vi "Lex Text-{} Unescaped Variable.vi"(8 "Error In":errorcluster) -> (0 "Error Out":errorcluster)   [LabVIEW 2018, in "Tests.lvlib" / "Lexer.lvlib"]
uses:
  Lexer.lvlib
  src/Toolkit/Low-Level/Tokens/Text/Text.lvclass
  src/Toolkit/Low-Level/Tokens/UnescapedVariable/UnescapedVariable.lvclass
  src/Toolkit/Low-Level/Tokens/Keyable/Keyable.lvclass/Keyable.ctl
  src/Toolkit/Low-Level/Tokens/Keyable/Read Key.vi
  src/Toolkit/Low-Level/Support/Lex String.vi
  <vilib>/Utility/LVClass/Get LV Class Name.vi
  src/Toolkit/Low-Level/Tokens/Contentable/Contentable.lvclass
  src/Toolkit/Low-Level/Tokens/Keyable/Keyable.lvclass
  <vilib>/addons/_JKI Toolkits/Caraya/classes/Test/Test.lvclass
  <vilib>/addons/_JKI Toolkits/Caraya/classes/Assert/Assert.lvclass
  src/Toolkit/Low-Level/Tokens/Abstract/Abstract.lvclass
  Tests.lvlib
  src/Toolkit/Toolkit.lvlib
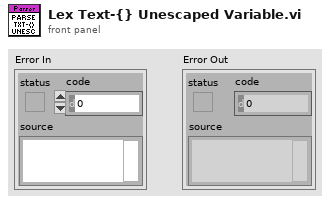
[diagram p1: front panel]
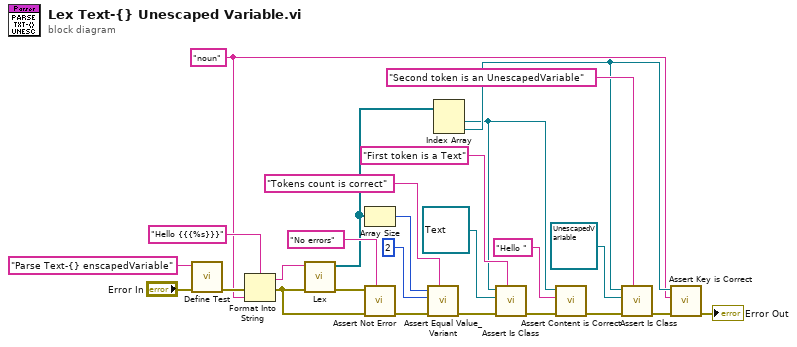
[diagram p0: block diagram]
diagram:
  w5 = "noun" ("String")
  n1 = call <vilib>:"Define Test.vi"("error in (no error)"="Error In", "Label (VI Title)"="Parse Text-{} enscapedVariable") -> ("error out"=w23:errorcluster)  [unwired: 9 in]
  n2 = Format Into String(format string="Hello {{{%s}}}", error in=w23, w5) -> (resulting string=w2:string, error out=w1:errorcluster)  [unwired: 1 in]
  n3 = call-poly "Lex.vi"("Error In"=w1, "Input"=w2) -> ("Error Out"=w24:errorcluster, "Tokens"=w16:refnum<class "Abstract.lvclass">[])  [unwired: 8 in]
  n4 = Array Size(array=w16) -> (size(s)=w19:i32)
  n5 = call <vilib>:"Assert Not Error.vi"("Label"="No errors", "error in (no error)"=w1, "Not Error?"=w24) -> ("error out"=w21:errorcluster)  [unwired: 8 in]
  n6 = call <vilib>:"Assert Equal Value_Variant.vi"("Label"="Tokens count is correct", "error in (no error)"=w21, "Y"=2 ("size(s)"), "X"=w19) -> ("error out"=w17:errorcluster)  [unwired: 7 in]
  n7 = Index Array(array=w16) -> (element #1=w4:refnum<class "Abstract.lvclass">, element #2=w7:refnum<class "Abstract.lvclass">)  [unwired: 2 in]
  n8 = call "Assert Is Class.vi"("Label"="First token is a Text", "Error In"=w17, "Expected"=refnum<class "Text.lvclass"> refnum ("Mustache.lvlib:Tokens.lvlib:Text.lvclass"), "Actual"=w4) -> ("Error Out"=w14:errorcluster)  [unwired: 7 in]
  n9 = call "Assert Content is Correct.vi"("Error In"=w14, "Expected"="Hello ", "Token"=w4) -> ("Error Out"=w13:errorcluster)  [unwired: 8 in]
  n10 = call "Assert Is Class.vi"("Label"="Second token is an UnescapedVariable", "Error In"=w13, "Expected"=refnum<class "UnescapedVariable.lvclass"> refnum ("Mustache.lvlib:Tokens.lvlib:UnescapedVariable.lvclass"), "Actual"=w7) -> ("Error Out"=w6:errorcluster)  [unwired: 7 in]
  n11 = call "Assert Key is Correct.vi"("Error In"=w6, "Expected"=w5, "Token"=w7) -> ("Error Out"=→"Error Out":errorcluster)  [unwired: 8 in]
